vi "Init.vi"(8 "error in (no error)":errorcluster, 10 "Topic":string, 11 "Pub Sub Message Channel in":refnum<class "Pub Sub Message Channel.lvclass">) -> (0 "error out":errorcluster, 3 "Pub Sub Message Channel out":refnum<class "Pub Sub Message Channel.lvclass">)   [LabVIEW 2020, in "Actor Pub Sub Channels.lvlib" / "Pub Sub Message Channel.lvclass"]
uses:
  Pub Sub Message Channel.lvclass
  <vilib>/ActorFramework/Message Enqueuer/Message Enqueuer.lvclass
  Pub Sub Message Channel.lvclass/Pub Sub Message Channel.ctl
  <vilib>/ActorFramework/Message Queue/Message Queue.lvclass
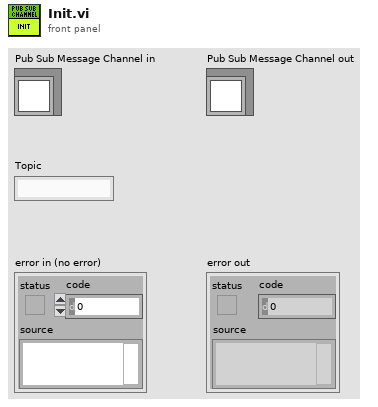
[diagram p1: front panel]
types:
  T1 = map{refnum<class "Message Enqueuer.lvclass">, string}
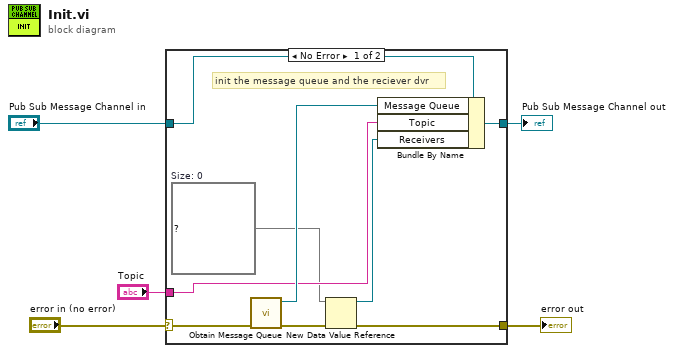
[diagram p0: block diagram]
diagram:
  n1 = case shown="No Error" "error in (no error)" {
    selector: "error in (no error)" -> [w13 w16]
    tunnel: [w7 w16] -> w4
    tunnel: [w12 w15] -> w2
    tunnel: "Pub Sub Message Channel in" -> [w14 w15]
    tunnel: "Topic" -> [w10 _]
    frame No Error {
      w6 = T1 {}  # Size: 0
      # "init the message queue and the reciever dvr"
      n2 = call <vilib>:"Obtain Message Queue.vi"("error in (no error)"=w13) -> ("error out"=w8:errorcluster, "Message Queue"=w11:refnum<class "Message Queue.lvclass">)  [unwired: 9 in]
      n3 = New Data Value Reference(data value=w6, error in=w8) -> (data value reference=w9:refnum<data-value>, error out=w7:errorcluster)
      n4 = Bundle By Name(cluster=w14, "Message Queue"=w11, "Topic"=w10, "Receivers"=w9) -> (w12:refnum<class "Pub Sub Message Channel.lvclass">)
    }
    frame Error {
    }
  }
  "error out" <- w4
  "Pub Sub Message Channel out" <- w2
